vi "FlipFlop.vi"(1 "Reset":bool, 2 "Set":bool) -> (0 "Ouput":bool)   [LabVIEW 2019]
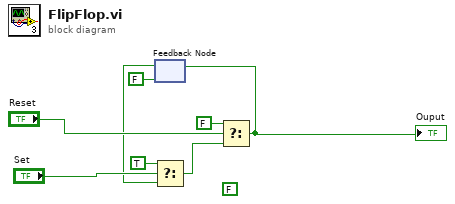
[diagram p0: block diagram]
diagram:
  (unwired) FALSE
  n1 = feedback #1(FALSE ("f")) -> (w4:bool)
  n2 = Select(t=TRUE, s="Set", f=w4) -> (s? t:f=w2:bool)
  n3 = Select(t=FALSE, s="Reset", f=w2) -> (s? t:f=w6:bool)
  "Ouput" <- w6
  n4 = feedback-in #1(w6) -> ()
